vi "Main.vi"(7 "sweep rate, /min":dbl=0.2, 8 "sweep to:":dbl=4.0, 9 "sweep":T8(radio)=enum."2636a_smub") -> ()   [LabVIEW 2021] (continued)
                      # "we are  measuring 2182A 3 channel 1 (2182A_3_ch1)"
                      n2137 = local read "2182A 3 addr"() -> (w2872:u8)
                      n2138 = Number To Decimal String(number=w2872) -> (decimal integer string=w2871:string)  [unwired: 1 in]
                      n2139 = GPIB Write(0:w2871, 1:":SENSe:DATA:FRES?") -> (6:w2876:errorcluster)  [unwired: 3 in, 1 out]
                      n2140 = GPIB Read(0:w2871, 1:200, 3:w2876) -> (5:w2870:string)  [unwired: 2 in, 2 out]
                      n2141 = Fract/Exp String To Number(string=w2870) -> (number=w2874:dbl)  [unwired: 3 in, 1 out]
                      n2142 = Build Array (concatenate)(w2878, w2874) -> (w2877:dbl[])
                    }
                  }
                  n2143 = property on="data" class="Arr (strict)"("Value"=w2868) -> ()  [unwired: 2 in, 2 out]
                }
                frame #21 {
                  # "check if 2nd channel \non Keithley 2182A 3\nis to be measured"
                  n2144 = property on="data" class="Arr (strict)"() -> ("Value"=w2880:dbl[])  [unwired: 2 in, 2 out]
                  n2145 = local read "2182A 3 ch2"() -> (w2879:bool)
                  n2146 = case shown="True" w2879 {
                    tunnel: w2880 -> [w2882 w2895]
                    tunnel: [w2882 w2894] -> w2881
                    frame False {
                      # "we are not measuring 2182A 3 channel 2 (2182A_3_ch2)"
                    }
                    frame True {
                      # "switching to channel 2 and then\nback to channel 1"
                      # "we are  measuring 2182A 3 channel 2 (2182A_3_ch2)"
                      n2147 = local read "2182A 3 addr"() -> (w2889:u8)
                      n2148 = Number To Decimal String(number=w2889) -> (decimal integer string=w2884:string)  [unwired: 1 in]
                      n2149 = GPIB Write(0:w2884, 1:":SENSe:CHAN 2") -> (6:w2886:errorcluster)  [unwired: 3 in, 1 out]
                      n2150 = GPIB Write(0:w2884, 1:":SENSe:DATA:FRES?", 3:w2886) -> (6:w2893:errorcluster)  [unwired: 2 in, 1 out]
                      n2151 = GPIB Read(0:w2884, 1:200, 3:w2893) -> (5:w2888:string, 7:w2885:errorcluster)  [unwired: 2 in, 1 out]
                      n2152 = GPIB Write(0:w2884, 1:":SENSe:CHAN 1", 3:w2885) -> ()  [unwired: 2 in, 2 out]
                      n2153 = Fract/Exp String To Number(string=w2888) -> (number=w2891:dbl)  [unwired: 3 in, 1 out]
                      n2154 = Build Array (concatenate)(w2895, w2891) -> (w2894:dbl[])
                    }
                  }
                  n2155 = property on="data" class="Arr (strict)"("Value"=w2881) -> ()  [unwired: 2 in, 2 out]
                }
                frame #22 {
                  # "check if 1st channel \non Keithley 2182A 4\nis to be measured"
                  n2156 = property on="data" class="Arr (strict)"() -> ("Value"=w2897:dbl[])  [unwired: 2 in, 2 out]
                  n2157 = local read "2182A 4 ch1"() -> (w2896:bool)
                  n2158 = case shown="True" w2896 {
                    tunnel: w2897 -> [w2899 w2908]
                    tunnel: [w2899 w2907] -> w2898
                    frame False {
                      # "we are not measuring 2182A 4 channel 1 (2182A_4_ch1)"
                    }
                    frame True {
                      # "we are  measuring 2182A 4 channel 1 (2182A_4_ch1)"
                      n2159 = local read "2182A 4 addr"() -> (w2902:u8)
                      n2160 = Number To Decimal String(number=w2902) -> (decimal integer string=w2901:string)  [unwired: 1 in]
                      n2161 = GPIB Write(0:w2901, 1:":SENSe:DATA:FRES?") -> (6:w2906:errorcluster)  [unwired: 3 in, 1 out]
                      n2162 = GPIB Read(0:w2901, 1:200, 3:w2906) -> (5:w2900:string)  [unwired: 2 in, 2 out]
                      n2163 = Fract/Exp String To Number(string=w2900) -> (number=w2904:dbl)  [unwired: 3 in, 1 out]
                      n2164 = Build Array (concatenate)(w2908, w2904) -> (w2907:dbl[])
                    }
                  }
                  n2165 = property on="data" class="Arr (strict)"("Value"=w2898) -> ()  [unwired: 2 in, 2 out]
                }
                frame #23 {
                  # "check if 2nd channel \non Keithley 2182A 4\nis to be measured"
                  n2166 = property on="data" class="Arr (strict)"() -> ("Value"=w2910:dbl[])  [unwired: 2 in, 2 out]
                  n2167 = local read "2182A 4 ch2"() -> (w2909:bool)
                  n2168 = case shown="False" w2909 {
                    tunnel: w2910 -> [w2912 w2925]
                    tunnel: [w2912 w2924] -> w2911
                    frame False {
                      # "we are not measuring 2182A 4 channel 2 (2182A_4_ch2)"
                    }
                    frame True {
                      # "switching to channel 2 and then\nback to channel 1"
                      # "we are  measuring 2182A 4 channel 2 (2182A_4_ch2)"
                      n2169 = local read "2182A 4 addr"() -> (w2919:u8)
                      n2170 = Number To Decimal String(number=w2919) -> (decimal integer string=w2914:string)  [unwired: 1 in]
                      n2171 = GPIB Write(0:w2914, 1:":SENSe:CHAN 2") -> (6:w2916:errorcluster)  [unwired: 3 in, 1 out]
                      n2172 = GPIB Write(0:w2914, 1:":SENSe:DATA:FRES?", 3:w2916) -> (6:w2923:errorcluster)  [unwired: 2 in, 1 out]
                      n2173 = GPIB Read(0:w2914, 1:200, 3:w2923) -> (5:w2918:string, 7:w2915:errorcluster)  [unwired: 2 in, 1 out]
                      n2174 = GPIB Write(0:w2914, 1:":SENSe:CHAN 1", 3:w2915) -> ()  [unwired: 2 in, 2 out]
                      n2175 = Fract/Exp String To Number(string=w2918) -> (number=w2921:dbl)  [unwired: 3 in, 1 out]
                      n2176 = Build Array (concatenate)(w2925, w2921) -> (w2924:dbl[])
                    }
                  }
                  n2177 = property on="data" class="Arr (strict)"("Value"=w2911) -> ()  [unwired: 2 in, 2 out]
                }
                frame #24 {
                  # "check if voltage on\nKeithley 2636A smua\nis to be measured"
                  n2178 = local read "2636A smua meas v"() -> (w2926:bool)
                  n2179 = property on="data" class="Arr (strict)"() -> ("Value"=w2927:dbl[])  [unwired: 2 in, 2 out]
                  n2180 = case shown="True" w2926 {
                    tunnel: w2927 -> [w2929 w2935]
                    tunnel: [w2929 w2934] -> w2928
                    frame False {
                      # "we are not measuring voltage on 2636A smua (2636A_smua_v)"
                    }
                    frame True {
                      # "we are  measuring voltage on 2636A smua (2636A_smua_v)"
                      n2181 = local read "2614A addr"() -> (w2930:refnum<visa-resource-name>)
                      n2182 = call "SinglePointMeasurement.vi"("Measure"=Measure."Voltage", "Channel"=Channel."a", "VISA resource name 2"=w2930) -> ("Measuremet"=w2932:dbl)  [unwired: 3 in, 4 out]
                      n2183 = Build Array (concatenate)(w2935, w2932) -> (w2934:dbl[])
                    }
                  }
                  n2184 = property on="data" class="Arr (strict)"("Value"=w2928) -> ()  [unwired: 2 in, 2 out]
                }
                frame #25 {
                  # "check if current on\nKeithley 2636A smua\nis to be measured"
                  n2185 = local read "2636A smua meas i"() -> (w2936:bool)
                  n2186 = property on="data" class="Arr (strict)"() -> ("Value"=w2937:dbl[])  [unwired: 2 in, 2 out]
                  n2187 = case shown="True" w2936 {
                    tunnel: w2937 -> [w2939 w2942]
                    tunnel: [w2939 w2941] -> w2938
                    frame False {
                      # "we are not measuring current on 2636A smua (2636A_smua_i)"
                    }
                    frame True {
                      # "we are  measuring current on 2636A smua (2636A_smua_i)"
                      n2188 = stacked-sequence {
                        tunnel: [_ w2951] -> w2940
                        frame #0 {
                          n2189 = local read "auto\nrange A"() -> (w2946:bool)
                          n2190 = local read "2614A addr"() -> (w2949:refnum<visa-resource-name>)
                          n2191 = Select(t="smua.AUTORANGE_ON", s=w2946, f="smua.AUTORANGE_OFF") -> (s? t:f=w2944:string)
                          n2192 = Concatenate Strings("smua.measure.autorangei = ", w2944) -> (w2943:string)
                          n2193 = VISA Write(VISA resource name=w2949, write buffer=w2943) -> ()  [unwired: 1 in, 3 out]
                        }
                        frame #1 {
                          n2194 = local read "2614A addr"() -> (w2953:refnum<visa-resource-name>)
                          n2195 = call "SinglePointMeasurement.vi"("Measure"=Measure."Current", "Channel"=Channel."a", "VISA resource name 2"=w2953) -> ("Measuremet"=w2951:dbl)  [unwired: 3 in, 4 out]
                        }
                      }
                      n2196 = Build Array (concatenate)(w2942, w2940) -> (w2941:dbl[])
                    }
                  }
                  n2197 = property on="data" class="Arr (strict)"("Value"=w2938) -> ()  [unwired: 2 in, 2 out]
                }
                frame #26 {
                  # "check if voltage on\nKeithley 2636A smub\nis to be measured"
                  n2198 = local read "2636A smub meas v"() -> (w2954:bool)
                  n2199 = property on="data" class="Arr (strict)"() -> ("Value"=w2955:dbl[])  [unwired: 2 in, 2 out]
                  n2200 = case shown="True" w2954 {
                    tunnel: w2955 -> [w2957 w2963]
                    tunnel: [w2957 w2962] -> w2956
                    frame False {
                      # "we are not measuring voltage on 2636A smub (2636A_smub_v)"
                    }
                    frame True {
                      # "we are  measuring voltage on 2636A smub (2636A_smub_v)"
                      n2201 = local read "2614A addr"() -> (w2961:refnum<visa-resource-name>)
                      n2202 = call "SinglePointMeasurement.vi"("Measure"=Measure."Voltage", "Channel"=Channel."b", "VISA resource name 2"=w2961) -> ("Measuremet"=w2959:dbl)  [unwired: 3 in, 4 out]
                      n2203 = Build Array (concatenate)(w2963, w2959) -> (w2962:dbl[])
                    }
                  }
                  n2204 = property on="data" class="Arr (strict)"("Value"=w2956) -> ()  [unwired: 2 in, 2 out]
                }
                frame #27 {
                  # "check if current on\nKeithley 2636A smub\nis to be measured"
                  n2205 = local read "2636A smub meas i"() -> (w2964:bool)
                  n2206 = property on="data" class="Arr (strict)"() -> ("Value"=w2965:dbl[])  [unwired: 2 in, 2 out]
                  n2207 = case shown="True" w2964 {
                    tunnel: w2965 -> [w2967 w2970]
                    tunnel: [w2967 w2969] -> w2966
                    frame False {
                      # "we are not measuring current on 2636A smub (2636A_smub_i)"
                    }
                    frame True {
                      # "we are  measuring current on 2636A smub (2636A_smub_i)"
                      n2208 = stacked-sequence {
                        tunnel: [_ w2979] -> w2968
                        frame #0 {
                          n2209 = local read "auto\nrange B"() -> (w2974:bool)
                          n2210 = local read "2614A addr"() -> (w2977:refnum<visa-resource-name>)
                          n2211 = Select(t="smub.AUTORANGE_ON", s=w2974, f="smub.AUTORANGE_OFF") -> (s? t:f=w2972:string)
                          n2212 = Concatenate Strings("smub.measure.autorangei = ", w2972) -> (w2971:string)
                          n2213 = VISA Write(VISA resource name=w2977, write buffer=w2971) -> ()  [unwired: 1 in, 3 out]
                        }
                        frame #1 {
                          n2214 = local read "2614A addr"() -> (w2981:refnum<visa-resource-name>)
                          n2215 = call "SinglePointMeasurement.vi"("Measure"=Measure."Current", "Channel"=Channel."b", "VISA resource name 2"=w2981) -> ("Measuremet"=w2979:dbl)  [unwired: 3 in, 4 out]
                        }
                      }
                      n2216 = Build Array (concatenate)(w2970, w2968) -> (w2969:dbl[])
                    }
                  }
                  n2217 = property on="data" class="Arr (strict)"("Value"=w2966) -> ()  [unwired: 2 in, 2 out]
                }
                frame #28 {
                  # "check if time\nis to be measured"
                  n2218 = property on="data" class="Arr (strict)"() -> ("Value"=w2984:dbl[])  [unwired: 2 in, 2 out]
                  n2219 = local read "measure time"() -> (w2983:bool)
                  n2220 = case shown="True" w2983 {
                    tunnel: w2984 -> [w2986 w2992]
                    tunnel: [w2986 w2991] -> w2985
                    tunnel: w2982 -> [_ w2989]
                    frame False {
                      # "we are not measuring time"
                    }
                    frame True {
                      # "seconds from the beginning of month"
                      # "we are  measuring time"
                      n2221 = call "timeInSeconds.vi"() -> ("Numeric"=w2990:dbl, "current time"=w2987:timestamp)  [unwired: 2 in]
                      n2222 = property on="current time" class="AbsTime (strict)"("Value"=w2987) -> ()  [unwired: 2 in, 2 out]
                      n2223 = Subtract(x=w2990, y=w2989) -> (x-y=w2988:dbl)
                      n2224 = Build Array (concatenate)(w2992, w2988) -> (w2991:dbl[])
                    }
                  }
                  n2225 = property on="data" class="Arr (strict)"("Value"=w2985) -> ()  [unwired: 2 in, 2 out]
                }
                frame #29 {
                  n2226 = local read "MagnetField"() -> (w2993:bool)
                  n2227 = property on="data" class="Arr (strict)"() -> ("Value"=w2994:dbl[])  [unwired: 2 in, 2 out]
                  n2228 = case shown="True" w2993 {
                    tunnel: w2994 -> [w2996 w2999]
                    tunnel: [w2996 w2998] -> w2995
                    frame False {
                      # "we are not Measuring magnetic field on IPS120-0"
                    }
                    frame True {
                      # "Measure magnetic field on Teslatron_iPS_Field"
                      n2229 = call "TRITON_Read Field.vi"() -> ("Measurement"=w2997:dbl)  [unwired: 2 in, 1 out]
                      n2230 = Build Array (concatenate)(w2999, w2997) -> (w2998:dbl[])
                    }
                  }
                  n2231 = property on="data" class="Arr (strict)"("Value"=w2995) -> ()  [unwired: 2 in, 2 out]
                }
                frame #30 {
                  n2232 = property on="data" class="Arr (strict)"() -> ("Value"=w3001:dbl[])  [unwired: 2 in, 2 out]
                  n2233 = property on="Magnet_T" class="Bool (strict)"() -> ("Value"=w3000:bool)  [unwired: 2 in, 2 out]
                  n2234 = case shown="True" w3000 {
                    tunnel: w3001 -> [w3003 w3007]
                    tunnel: [w3003 w3006] -> w3002
                    frame False {
                      # "we are not Measuring magnetic field on IPS120-0"
                    }
                    frame True {
                      # "Measure magnetic_T on Teslatron"
                      n2235 = call "TRITON_Read Temperature.vi"("Channel"=13 ("Ch2")) -> ("Measuremet"=w3004:dbl)  [unwired: 1 in, 1 out]
                      n2236 = Build Array (concatenate)(w3007, w3004) -> (w3006:dbl[])
                    }
                  }
                  n2237 = property on="data" class="Arr (strict)"("Value"=w3002) -> ()  [unwired: 2 in, 2 out]
                }
                frame #31 {
                  n2238 = property on="data" class="Arr (strict)"() -> ("Value"=w3009:dbl[])  [unwired: 2 in, 2 out]
                  n2239 = property on="PT1" class="Bool (strict)"() -> ("Value"=w3008:bool)  [unwired: 2 in, 2 out]
                  n2240 = case shown="True" w3008 {
                    tunnel: w3009 -> [w3011 w3015]
                    tunnel: [w3011 w3014] -> w3010
                    frame False {
                      # "we are not Measuring magnetic field on IPS120-0"
                    }
                    frame True {
                      # "Measure  SH_T on Teslatron"
                      n2241 = call "TRITON_Read Temperature.vi"("Channel"=7 ("Ch2")) -> ("Measuremet"=w3012:dbl)  [unwired: 1 in, 1 out]
                      n2242 = Build Array (concatenate)(w3015, w3012) -> (w3014:dbl[])
                    }
                  }
                  n2243 = property on="data" class="Arr (strict)"("Value"=w3010) -> ()  [unwired: 2 in, 2 out]
                }
                frame #32 {
                  # "check if current \non 2461 SouceMeter\nis to be measured"
                  n2244 = property on="data" class="Arr (strict)"() -> ("Value"=w3017:dbl[])  [unwired: 2 in, 2 out]
                  n2245 = property on="MC_RuO2" class="Bool (strict)"() -> ("Value"=w3016:bool)  [unwired: 2 in, 2 out]
                  n2246 = case shown="True" w3016 {
                    tunnel: w3017 -> [w3019 w3023]
                    tunnel: [w3019 w3022] -> w3018
                    frame False {
                      # "we are not measuring 2461, voltage (2461_meas_v)"
                    }
                    frame True {
                      # "we are  measuring 2461, voltage (2461_meas_v)"
                      n2247 = call "TRITON_Read Temperature.vi"("Channel"=8 ("Ch2")) -> ("Measuremet"=w3020:dbl)  [unwired: 1 in, 1 out]
                      n2248 = Build Array (concatenate)(w3023, w3020) -> (w3022:dbl[])
                    }
                  }
                  n2249 = property on="data" class="Arr (strict)"("Value"=w3018) -> ()  [unwired: 2 in, 2 out]
                }
                frame #33 {
                  # "check if current \non 2461 SouceMeter\nis to be measured"
                  n2250 = property on="data" class="Arr (strict)"() -> ("Value"=w3025:dbl[])  [unwired: 2 in, 2 out]
                  n2251 = property on="Still" class="Bool (strict)"() -> ("Value"=w3024:bool)  [unwired: 2 in, 2 out]
                  n2252 = case shown="True" w3024 {
                    tunnel: w3025 -> [w3027 w3031]
                    tunnel: [w3027 w3030] -> w3026
                    frame False {
                      # "we are not measuring 2461, voltage (2461_meas_v)"
                    }
                    frame True {
                      # "we are  measuring 2461, voltage (2461_meas_v)"
                      n2253 = call "TRITON_Read Temperature.vi"("Channel"=3 ("Ch2")) -> ("Measuremet"=w3028:dbl)  [unwired: 1 in, 1 out]
                      n2254 = Build Array (concatenate)(w3031, w3028) -> (w3030:dbl[])
                    }
                  }
                  n2255 = property on="data" class="Arr (strict)"("Value"=w3026) -> ()  [unwired: 2 in, 2 out]
                }
                frame #34 {
                  # "check if current \non 2461 SouceMeter\nis to be measured"
                  n2256 = property on="data" class="Arr (strict)"() -> ("Value"=w3033:dbl[])  [unwired: 2 in, 2 out]
                  n2257 = property on="Cold_Plate" class="Bool (strict)"() -> ("Value"=w3032:bool)  [unwired: 2 in, 2 out]
                  n2258 = case shown="True" w3032 {
                    tunnel: w3033 -> [w3035 w3039]
                    tunnel: [w3035 w3038] -> w3034
                    frame False {
                      # "we are not measuring 2461, voltage (2461_meas_v)"
                    }
                    frame True {
                      # "we are  measuring 2461, voltage (2461_meas_v)"
                      n2259 = call "TRITON_Read Temperature.vi"("Channel"=4 ("Ch2")) -> ("Measuremet"=w3036:dbl)  [unwired: 1 in, 1 out]
                      n2260 = Build Array (concatenate)(w3039, w3036) -> (w3038:dbl[])
                    }
                  }
                  n2261 = property on="data" class="Arr (strict)"("Value"=w3034) -> ()  [unwired: 2 in, 2 out]
                }
                frame #35 {
                  # "check if current \non 2461 SouceMeter\nis to be measured"
                  n2262 = property on="data" class="Arr (strict)"() -> ("Value"=w3041:dbl[])  [unwired: 2 in, 2 out]
                  n2263 = property on="PT2" class="Bool (strict)"() -> ("Value"=w3040:bool)  [unwired: 2 in, 2 out]
                  n2264 = case shown="True" w3040 {
                    tunnel: w3041 -> [w3043 w3047]
                    tunnel: [w3043 w3046] -> w3042
                    frame False {
                      # "we are not measuring 2461, voltage (2461_meas_v)"
                    }
                    frame True {
                      # "we are  measuring 2461, voltage (2461_meas_v)"
                      n2265 = call "TRITON_Read Temperature.vi"("Channel"=2 ("Ch2")) -> ("Measuremet"=w3044:dbl)  [unwired: 1 in, 1 out]
                      n2266 = Build Array (concatenate)(w3047, w3044) -> (w3046:dbl[])
                    }
                  }
                  n2267 = property on="data" class="Arr (strict)"("Value"=w3042) -> ()  [unwired: 2 in, 2 out]
                }
                frame #36 {
                  # "check if current \non 2461 SouceMeter\nis to be measured"
                  n2268 = property on="data" class="Arr (strict)"() -> ("Value"=w3049:dbl[])  [unwired: 2 in, 2 out]
                  n2269 = property on="MC_Cernox" class="Bool (strict)"() -> ("Value"=w3048:bool)  [unwired: 2 in, 2 out]
                  n2270 = case shown="True" w3048 {
                    tunnel: w3049 -> [w3051 w3055]
                    tunnel: [w3051 w3054] -> w3050
                    frame False {
                      # "we are not measuring 2461, voltage (2461_meas_v)"
                    }
                    frame True {
                      # "we are  measuring 2461, voltage (2461_meas_v)"
                      n2271 = call "TRITON_Read Temperature.vi"("Channel"=5 ("Ch2")) -> ("Measuremet"=w3052:dbl)  [unwired: 1 in, 1 out]
                      n2272 = Build Array (concatenate)(w3055, w3052) -> (w3054:dbl[])
                    }
                  }
                  n2273 = property on="data" class="Arr (strict)"("Value"=w3050) -> ()  [unwired: 2 in, 2 out]
                }
                frame #37 {
                  # "check if current \non 2461 SouceMeter\nis to be measured"
                  n2274 = property on="2461_meas_v" class="Bool (strict)"() -> ("Value"=w3056:bool)  [unwired: 2 in, 2 out]
                  n2275 = property on="data" class="Arr (strict)"() -> ("Value"=w3057:dbl[])  [unwired: 2 in, 2 out]
                  n2276 = case shown="True" w3056 {
                    tunnel: w3057 -> [w3059 w3064]
                    tunnel: [w3059 w3063] -> w3058
                    frame False {
                      # "we are not measuring 2461, voltage (2461_meas_v)"
                    }
                    frame True {
                      # "we are  measuring 2461, voltage (2461_meas_v)"
                      n2277 = property on="2461_addr_sweep" class="VISAName"() -> ("Value"=w3061:refnum<visa-resource-name>)  [unwired: 2 in, 2 out]
                      n2278 = call <instrlib>:"Read (Single Point).vi"("VISA resource name"=w3061) -> ("Data out"=w3060:string)  [unwired: 12 in, 2 out]
                      n2279 = Fract/Exp String To Number(string=w3060) -> (number=w3062:dbl)  [unwired: 3 in, 1 out]
                      n2280 = Build Array (concatenate)(w3064, w3062) -> (w3063:dbl[])
                    }
                  }
                  n2281 = property on="data" class="Arr (strict)"("Value"=w3058) -> ()  [unwired: 2 in, 2 out]
                }
                frame #38 {
                  # "check if current \non 2461 SouceMeter\nis to be measured"
                  n2282 = property on="2461_meas_i" class="Bool (strict)"() -> ("Value"=w3065:bool)  [unwired: 2 in, 2 out]
                  n2283 = property on="data" class="Arr (strict)"() -> ("Value"=w3066:dbl[])  [unwired: 2 in, 2 out]
                  n2284 = case shown="True" w3065 {
                    tunnel: w3066 -> [w3068 w3072]
                    tunnel: [w3068 w3071] -> w3067
                    frame False {
                      # "we are not measuring 2461, voltage (2461_meas_v)"
                    }
                    frame True {
                      # "we are  measuring 2461, curent (2461_meas_i)"
                      n2285 = property on="2461_addr_sweep" class="VISAName"() -> ("Value"=w3070:refnum<visa-resource-name>)  [unwired: 2 in, 2 out]
                      n2286 = call <instrlib>:"Get Source Level.vi"("VISA resource name"=w3070) -> ("Current Level Out"=w3069:dbl)  [unwired: 7 in, 3 out]
                      n2287 = Build Array (concatenate)(w3072, w3069) -> (w3071:dbl[])
                    }
                  }
                  n2288 = property on="data" class="Arr (strict)"("Value"=w3067) -> ()  [unwired: 2 in, 2 out]
                }
                frame #39 {
                  # "Record Step Value \nif it is mapping"
                  n2289 = property on="Linetrace or Mapping?" class="Bool (strict)"() -> ("Value"=w3074:bool)  [unwired: 2 in, 2 out]
                  n2290 = property on="data" class="Arr (strict)"() -> ("Value"=w3075:dbl[])  [unwired: 2 in, 2 out]
                  n2291 = case shown="True" w3074 {
                    tunnel: w3075 -> [w3076 w3079]
                    tunnel: [w3076 w3078] -> w3073
                    frame False {
                      # "We are not recording Step Value if it is linetrace"
                    }
                    frame True {
                      # "We are recording Step Value if it is mapping"
                      n2292 = property on="Current Step Value" class="DigNum (strict)"() -> ("Value"=w3077:dbl)  [unwired: 2 in, 2 out]
                      n2293 = Build Array (concatenate)(w3079, w3077) -> (w3078:dbl[])
                    }
                  }
                  n2294 = property on="data" class="Arr (strict)"("Value"=w3073) -> ()  [unwired: 2 in, 2 out]
                }
                frame #40 {
                  # "Record Step Value \nif it is mapping"
                  n2295 = property on="HyperLoop" class="Bool (strict)"() -> ("Value"=w3080:bool)  [unwired: 2 in, 2 out]
                  n2296 = property on="data" class="Arr (strict)"() -> ("Value"=w3082:dbl[])  [unwired: 2 in, 2 out]
                  n2297 = case shown="True" w3080 {
                    tunnel: w3082 -> [w3083 w3086]
                    tunnel: [w3083 w3085] -> w3081
                    frame False {
                      # "We are not recording Step Value if it is linetrace"
                    }
                    frame True {
                      # "We are recording Step Value if it is mapping"
                      n2298 = property on="Current Hyper Value" class="DigNum (strict)"() -> ("Value"=w3084:dbl)  [unwired: 2 in, 2 out]
                      n2299 = Build Array (concatenate)(w3086, w3084) -> (w3085:dbl[])
                    }
                  }
                  n2300 = property on="data" class="Arr (strict)"("Value"=w3081) -> ()  [unwired: 2 in, 2 out]
                }
                frame #41 {
                  # "Record Step Value \nif it is mapping"
                  n2301 = property on="SuperHyper" class="Bool (strict)"() -> ("Value"=w3087:bool)  [unwired: 2 in, 2 out]
                  n2302 = property on="data" class="Arr (strict)"() -> ("Value"=w3089:dbl[])  [unwired: 2 in, 2 out]
                  n2303 = case shown="True" w3087 {
                    tunnel: w3089 -> [w3090 w3093]
                    tunnel: [w3090 w3092] -> w3088
                    frame False {
                      # "We are not recording Step Value if it is linetrace"
                    }
                    frame True {
                      # "We are recording SuperHyper_step if it is mapping"
                      n2304 = property on="Current SuperHyper Value" class="DigNum (strict)"() -> ("Value"=w3091:dbl)  [unwired: 2 in, 2 out]
                      n2305 = Build Array (concatenate)(w3093, w3091) -> (w3092:dbl[])
                    }
                  }
                  n2306 = property on="data" class="Arr (strict)"("Value"=w3088) -> ()  [unwired: 2 in, 2 out]
                }
                frame #42 {
                  # "Measure MFLI_V if \nit is checked"
                  n2307 = property on="MFLI1_d0" class="Bool (strict)"() -> ("Value"=w3094:bool)  [unwired: 2 in, 2 out]
                  n2308 = property on="data" class="Arr (strict)"() -> ("Value"=w3096:dbl[])  [unwired: 2 in, 2 out]
                  n2309 = case shown="True" w3094 {
                    tunnel: w3096 -> [w3097 w3102]
                    tunnel: [w3097 w3101] -> w3095
                    frame False {
                      # "We are not recording Step Value if it is linetrace"
                    }
                    frame True {
                      n2310 = flat-sequence {
                        tunnel: [w3106] -> w3100
                        tunnel: [w3105] -> w3099
                        tunnel: [w3104] -> w3098
                        frame #0 {
                          n2311 = property on="HandleOut" class="Clust (strict)"() -> ("Value"=w3108:T1)  [unwired: 2 in, 2 out]
                          n2312 = call "MFLIcontrol.vi"("MFLI function"=MFLIcommand."measure XY on demod0", "handle in"=w3108) -> ("Demod Sample Out 2"=w3103:T20)  [unwired: 5 in, 4 out]
                          n2313 = Unbundle(w3103) -> ("X (Vrms)"=w3106:dbl, "Y (Vrms)"=w3105:dbl, "Freq (Hz)"=w3104:dbl)  [unwired: 6 out]
                        }
                      }
                      n2314 = Build Array (concatenate)(w3102, w3100, w3099, w3098) -> (w3101:dbl[])
                    }
                  }
                  n2315 = property on="data" class="Arr (strict)"("Value"=w3095) -> ()  [unwired: 2 in, 2 out]
                }
                frame #43 {
                  # "Measure MFLI_V if \nit is checked"
                  n2316 = property on="MFLI2_d0" class="Bool (strict)"() -> ("Value"=w3109:bool)  [unwired: 2 in, 2 out]
                  n2317 = property on="data" class="Arr (strict)"() -> ("Value"=w3111:dbl[])  [unwired: 2 in, 2 out]
                  n2318 = case shown="True" w3109 {
                    tunnel: w3111 -> [w3112 w3117]
                    tunnel: [w3112 w3116] -> w3110
                    frame False {
                      # "We are not recording Step Value if it is linetrace"
                    }
                    frame True {
                      n2319 = flat-sequence {
                        tunnel: [w3121] -> w3115
                        tunnel: [w3120] -> w3114
                        tunnel: [w3119] -> w3113
                        frame #0 {
                          n2320 = property on="HandleOut 2" class="Clust (strict)"() -> ("Value"=w3123:T21)  [unwired: 2 in, 2 out]
                          n2321 = call "MFLIcontrol.vi"("MFLI function"=MFLIcommand."measure XY on demod0", "handle in"=w3123) -> ("Demod Sample Out 2"=w3118:T20)  [unwired: 5 in, 4 out]
                          n2322 = Unbundle(w3118) -> ("X (Vrms)"=w3121:dbl, "Y (Vrms)"=w3120:dbl, "Freq (Hz)"=w3119:dbl)  [unwired: 6 out]
                        }
                      }
                      n2323 = Build Array (concatenate)(w3117, w3115, w3114, w3113) -> (w3116:dbl[])
                    }
                  }
                  n2324 = property on="data" class="Arr (strict)"("Value"=w3110) -> ()  [unwired: 2 in, 2 out]
                }
                frame #44 {
                  # "Measure MFLI_V if \nit is checked"
                  n2325 = property on="MFLI3_d0" class="Bool (strict)"() -> ("Value"=w3124:bool)  [unwired: 2 in, 2 out]
                  n2326 = property on="data" class="Arr (strict)"() -> ("Value"=w3126:dbl[])  [unwired: 2 in, 2 out]
                  n2327 = case shown="True" w3124 {
                    tunnel: w3126 -> [w3127 w3132]
                    tunnel: [w3127 w3131] -> w3125
                    frame False {
                      # "We are not recording Step Value if it is linetrace"
                    }
                    frame True {
                      n2328 = flat-sequence {
                        tunnel: [w3136] -> w3130
                        tunnel: [w3135] -> w3129
                        tunnel: [w3134] -> w3128
                        frame #0 {
                          n2329 = property on="HandleOut 3" class="Clust (strict)"() -> ("Value"=w3138:T21)  [unwired: 2 in, 2 out]
                          n2330 = call "MFLIcontrol.vi"("MFLI function"=MFLIcommand."measure XY on demod0", "handle in"=w3138) -> ("Demod Sample Out 2"=w3133:T20)  [unwired: 5 in, 4 out]
                          n2331 = Unbundle(w3133) -> ("X (Vrms)"=w3136:dbl, "Y (Vrms)"=w3135:dbl, "Freq (Hz)"=w3134:dbl)  [unwired: 6 out]
                        }
                      }
                      n2332 = Build Array (concatenate)(w3132, w3130, w3129, w3128) -> (w3131:dbl[])
                    }
                  }
                  n2333 = property on="data" class="Arr (strict)"("Value"=w3125) -> ()  [unwired: 2 in, 2 out]
                }
                frame #45 {
                  # "Measure MFLI_V if \nit is checked"
                  n2334 = property on="MFLI4_d0" class="Bool (strict)"() -> ("Value"=w3139:bool)  [unwired: 2 in, 2 out]
                  n2335 = property on="data" class="Arr (strict)"() -> ("Value"=w3141:dbl[])  [unwired: 2 in, 2 out]
                  n2336 = case shown="True" w3139 {
                    tunnel: w3141 -> [w3142 w3147]
                    tunnel: [w3142 w3146] -> w3140
                    frame False {
                      # "We are not recording Step Value if it is linetrace"
                    }
                    frame True {
                      n2337 = flat-sequence {
                        tunnel: [w3151] -> w3145
                        tunnel: [w3150] -> w3144
                        tunnel: [w3149] -> w3143
                        frame #0 {
                          n2338 = property on="HandleOut 4" class="Clust (strict)"() -> ("Value"=w3153:T21)  [unwired: 2 in, 2 out]
                          n2339 = call "MFLIcontrol.vi"("MFLI function"=MFLIcommand."measure XY on demod0", "handle in"=w3153) -> ("Demod Sample Out 2"=w3148:T20)  [unwired: 5 in, 4 out]
                          n2340 = Unbundle(w3148) -> ("X (Vrms)"=w3151:dbl, "Y (Vrms)"=w3150:dbl, "Freq (Hz)"=w3149:dbl)  [unwired: 6 out]
                        }
                      }
                      n2341 = Build Array (concatenate)(w3147, w3145, w3144, w3143) -> (w3146:dbl[])
                    }
                  }
                  n2342 = property on="data" class="Arr (strict)"("Value"=w3140) -> ()  [unwired: 2 in, 2 out]
                }
                frame #46 {
                  # "Measure MFLI_I if \nit is checked"
                  n2343 = property on="MFLI1_d1" class="Bool (strict)"() -> ("Value"=w3154:bool)  [unwired: 2 in, 2 out]
                  n2344 = property on="data" class="Arr (strict)"() -> ("Value"=w3156:dbl[])  [unwired: 2 in, 2 out]
                  n2345 = case shown="True" w3154 {
                    tunnel: w3156 -> [w3157 w3162]
                    tunnel: [w3157 w3161] -> w3155
                    frame False {
                      # "We are not recording Step Value if it is linetrace"
                    }
                    frame True {
                      n2346 = flat-sequence {
                        tunnel: [w3165] -> w3160
                        tunnel: [w3164] -> w3159
                        tunnel: [w3163] -> w3158
                        frame #0 {
                          n2347 = property on="HandleOut" class="Clust (strict)"() -> ("Value"=w3168:T1)  [unwired: 2 in, 2 out]
                          n2348 = call "MFLIcontrol.vi"("MFLI function"=MFLIcommand."measure XY on demod1", "handle in"=w3168) -> ("Demod Sample Out 3"=w3166:T20)  [unwired: 5 in, 4 out]
                          n2349 = Unbundle(w3166) -> ("X (Vrms)"=w3165:dbl, "Y (Vrms)"=w3164:dbl, "Freq (Hz)"=w3163:dbl)  [unwired: 6 out]
                        }
                      }
                      n2350 = Build Array (concatenate)(w3162, w3160, w3159, w3158) -> (w3161:dbl[])
                    }
                  }
                  n2351 = property on="data" class="Arr (strict)"("Value"=w3155) -> ()  [unwired: 2 in, 2 out]
                }
                frame #47 {
                  # "Measure MFLI_I if \nit is checked"
                  n2352 = property on="MFLI2_d1" class="Bool (strict)"() -> ("Value"=w3169:bool)  [unwired: 2 in, 2 out]
                  n2353 = property on="data" class="Arr (strict)"() -> ("Value"=w3171:dbl[])  [unwired: 2 in, 2 out]
                  n2354 = case shown="True" w3169 {
                    tunnel: w3171 -> [w3172 w3177]
                    tunnel: [w3172 w3176] -> w3170
                    frame False {
                      # "We are not recording Step Value if it is linetrace"
                    }
                    frame True {
                      n2355 = flat-sequence {
                        tunnel: [w3180] -> w3175
                        tunnel: [w3179] -> w3174
                        tunnel: [w3178] -> w3173
                        frame #0 {
                          n2356 = property on="HandleOut 2" class="Clust (strict)"() -> ("Value"=w3183:T21)  [unwired: 2 in, 2 out]
                          n2357 = call "MFLIcontrol.vi"("MFLI function"=MFLIcommand."measure XY on demod1", "handle in"=w3183) -> ("Demod Sample Out 3"=w3181:T20)  [unwired: 5 in, 4 out]
                          n2358 = Unbundle(w3181) -> ("X (Vrms)"=w3180:dbl, "Y (Vrms)"=w3179:dbl, "Freq (Hz)"=w3178:dbl)  [unwired: 6 out]
                        }
                      }
                      n2359 = Build Array (concatenate)(w3177, w3175, w3174, w3173) -> (w3176:dbl[])
                    }
                  }
                  n2360 = property on="data" class="Arr (strict)"("Value"=w3170) -> ()  [unwired: 2 in, 2 out]
                }
                frame #48 {
                  # "Measure MFLI_I if \nit is checked"
                  n2361 = property on="MFLI3_d1" class="Bool (strict)"() -> ("Value"=w3184:bool)  [unwired: 2 in, 2 out]
                  n2362 = property on="data" class="Arr (strict)"() -> ("Value"=w3186:dbl[])  [unwired: 2 in, 2 out]
                  n2363 = case shown="True" w3184 {
                    tunnel: w3186 -> [w3187 w3192]
                    tunnel: [w3187 w3191] -> w3185
                    frame False {
                      # "We are not recording Step Value if it is linetrace"
                    }
                    frame True {
                      n2364 = flat-sequence {
                        tunnel: [w3195] -> w3190
                        tunnel: [w3194] -> w3189
                        tunnel: [w3193] -> w3188
                        frame #0 {
                          n2365 = property on="HandleOut 3" class="Clust (strict)"() -> ("Value"=w3198:T21)  [unwired: 2 in, 2 out]
                          n2366 = call "MFLIcontrol.vi"("MFLI function"=MFLIcommand."measure XY on demod1", "handle in"=w3198) -> ("Demod Sample Out 3"=w3196:T20)  [unwired: 5 in, 4 out]
                          n2367 = Unbundle(w3196) -> ("X (Vrms)"=w3195:dbl, "Y (Vrms)"=w3194:dbl, "Freq (Hz)"=w3193:dbl)  [unwired: 6 out]
                        }
                      }
                      n2368 = Build Array (concatenate)(w3192, w3190, w3189, w3188) -> (w3191:dbl[])
                    }
                  }
                  n2369 = property on="data" class="Arr (strict)"("Value"=w3185) -> ()  [unwired: 2 in, 2 out]
                }
                frame #49 {
                  # "Measure MFLI_I if \nit is checked"
                  n2370 = property on="MFLI4_d1" class="Bool (strict)"() -> ("Value"=w3199:bool)  [unwired: 2 in, 2 out]
                  n2371 = property on="data" class="Arr (strict)"() -> ("Value"=w3201:dbl[])  [unwired: 2 in, 2 out]
                  n2372 = case shown="True" w3199 {
                    tunnel: w3201 -> [w3202 w3207]
                    tunnel: [w3202 w3206] -> w3200
                    frame False {
                      # "We are not recording Step Value if it is linetrace"
                    }
                    frame True {
                      n2373 = flat-sequence {
                        tunnel: [w3210] -> w3205
                        tunnel: [w3209] -> w3204
                        tunnel: [w3208] -> w3203
                        frame #0 {
                          n2374 = property on="HandleOut 4" class="Clust (strict)"() -> ("Value"=w3213:T21)  [unwired: 2 in, 2 out]
                          n2375 = call "MFLIcontrol.vi"("MFLI function"=MFLIcommand."measure XY on demod1", "handle in"=w3213) -> ("Demod Sample Out 3"=w3211:T20)  [unwired: 5 in, 4 out]
                          n2376 = Unbundle(w3211) -> ("X (Vrms)"=w3210:dbl, "Y (Vrms)"=w3209:dbl, "Freq (Hz)"=w3208:dbl)  [unwired: 6 out]
                        }
                      }
                      n2377 = Build Array (concatenate)(w3207, w3205, w3204, w3203) -> (w3206:dbl[])
                    }
                  }
                  n2378 = property on="data" class="Arr (strict)"("Value"=w3200) -> ()  [unwired: 2 in, 2 out]
                }
                frame #50 {
                  # "Measure MFLI_I if \nit is checked"
                  n2379 = property on="MFLI1_d2" class="Bool (strict)"() -> ("Value"=w3214:bool)  [unwired: 2 in, 2 out]
                  n2380 = property on="data" class="Arr (strict)"() -> ("Value"=w3216:dbl[])  [unwired: 2 in, 2 out]
                  n2381 = case shown="True" w3214 {
                    tunnel: w3216 -> [w3217 w3222]
                    tunnel: [w3217 w3221] -> w3215
                    frame False {
                      # "We are not recording Step Value if it is linetrace"
                    }
                    frame True {
                      n2382 = flat-sequence {
                        tunnel: [w3225] -> w3220
                        tunnel: [w3224] -> w3219
                        tunnel: [w3223] -> w3218
                        frame #0 {
                          n2383 = property on="HandleOut" class="Clust (strict)"() -> ("Value"=w3228:T1)  [unwired: 2 in, 2 out]
                          n2384 = call "MFLIcontrol.vi"("MFLI function"=MFLIcommand."measure XY on demod2", "handle in"=w3228) -> ("Demod Sample Out 3"=w3226:T20)  [unwired: 5 in, 4 out]
                          n2385 = Unbundle(w3226) -> ("X (Vrms)"=w3225:dbl, "Y (Vrms)"=w3224:dbl, "Freq (Hz)"=w3223:dbl)  [unwired: 6 out]
                        }
                      }
                      n2386 = Build Array (concatenate)(w3222, w3220, w3219, w3218) -> (w3221:dbl[])
                    }
                  }
                  n2387 = property on="data" class="Arr (strict)"("Value"=w3215) -> ()  [unwired: 2 in, 2 out]
                }
                frame #51 {
                  # "Measure MFLI_I if \nit is checked"
                  n2388 = property on="MFLI2_d2" class="Bool (strict)"() -> ("Value"=w3229:bool)  [unwired: 2 in, 2 out]
                  n2389 = property on="data" class="Arr (strict)"() -> ("Value"=w3231:dbl[])  [unwired: 2 in, 2 out]
                  n2390 = case shown="True" w3229 {
                    tunnel: w3231 -> [w3232 w3237]
                    tunnel: [w3232 w3236] -> w3230
                    frame False {
                      # "We are not recording Step Value if it is linetrace"
                    }
                    frame True {
                      n2391 = flat-sequence {
                        tunnel: [w3240] -> w3235
                        tunnel: [w3239] -> w3234
                        tunnel: [w3238] -> w3233
                        frame #0 {
                          n2392 = property on="HandleOut 2" class="Clust (strict)"() -> ("Value"=w3243:T21)  [unwired: 2 in, 2 out]
                          n2393 = call "MFLIcontrol.vi"("MFLI function"=MFLIcommand."measure XY on demod2", "handle in"=w3243) -> ("Demod Sample Out 3"=w3241:T20)  [unwired: 5 in, 4 out]
                          n2394 = Unbundle(w3241) -> ("X (Vrms)"=w3240:dbl, "Y (Vrms)"=w3239:dbl, "Freq (Hz)"=w3238:dbl)  [unwired: 6 out]
                        }
                      }
                      n2395 = Build Array (concatenate)(w3237, w3235, w3234, w3233) -> (w3236:dbl[])
                    }
                  }
                  n2396 = property on="data" class="Arr (strict)"("Value"=w3230) -> ()  [unwired: 2 in, 2 out]
                }
                frame #52 {
                  # "Measure MFLI_I if \nit is checked"
                  n2397 = property on="MFLI3_d2" class="Bool (strict)"() -> ("Value"=w3244:bool)  [unwired: 2 in, 2 out]
                  n2398 = property on="data" class="Arr (strict)"() -> ("Value"=w3246:dbl[])  [unwired: 2 in, 2 out]
                  n2399 = case shown="True" w3244 {
                    tunnel: w3246 -> [w3247 w3252]
                    tunnel: [w3247 w3251] -> w3245
                    frame False {
                      # "We are not recording Step Value if it is linetrace"
                    }
                    frame True {
                      n2400 = flat-sequence {
                        tunnel: [w3255] -> w3250
                        tunnel: [w3254] -> w3249
                        tunnel: [w3253] -> w3248
                        frame #0 {
                          n2401 = property on="HandleOut 3" class="Clust (strict)"() -> ("Value"=w3258:T21)  [unwired: 2 in, 2 out]
                          n2402 = call "MFLIcontrol.vi"("MFLI function"=MFLIcommand."measure XY on demod2", "handle in"=w3258) -> ("Demod Sample Out 3"=w3256:T20)  [unwired: 5 in, 4 out]
                          n2403 = Unbundle(w3256) -> ("X (Vrms)"=w3255:dbl, "Y (Vrms)"=w3254:dbl, "Freq (Hz)"=w3253:dbl)  [unwired: 6 out]
                        }
                      }
                      n2404 = Build Array (concatenate)(w3252, w3250, w3249, w3248) -> (w3251:dbl[])
                    }
                  }
                  n2405 = property on="data" class="Arr (strict)"("Value"=w3245) -> ()  [unwired: 2 in, 2 out]
                }
                frame #53 {
                  # "Measure MFLI_I if \nit is checked"
                  n2406 = property on="MFLI4_d2" class="Bool (strict)"() -> ("Value"=w3259:bool)  [unwired: 2 in, 2 out]
                  n2407 = property on="data" class="Arr (strict)"() -> ("Value"=w3261:dbl[])  [unwired: 2 in, 2 out]
                  n2408 = case shown="True" w3259 {
                    tunnel: w3261 -> [w3262 w3267]
                    tunnel: [w3262 w3266] -> w3260
                    frame False {
                      # "We are not recording Step Value if it is linetrace"
                    }
                    frame True {
                      n2409 = flat-sequence {
                        tunnel: [w3270] -> w3265
                        tunnel: [w3269] -> w3264
                        tunnel: [w3268] -> w3263
                        frame #0 {
                          n2410 = property on="HandleOut 4" class="Clust (strict)"() -> ("Value"=w3273:T21)  [unwired: 2 in, 2 out]
                          n2411 = call "MFLIcontrol.vi"("MFLI function"=MFLIcommand."measure XY on demod2", "handle in"=w3273) -> ("Demod Sample Out 3"=w3271:T20)  [unwired: 5 in, 4 out]
                          n2412 = Unbundle(w3271) -> ("X (Vrms)"=w3270:dbl, "Y (Vrms)"=w3269:dbl, "Freq (Hz)"=w3268:dbl)  [unwired: 6 out]
                        }
                      }
                      n2413 = Build Array (concatenate)(w3267, w3265, w3264, w3263) -> (w3266:dbl[])
                    }
                  }
                  n2414 = property on="data" class="Arr (strict)"("Value"=w3260) -> ()  [unwired: 2 in, 2 out]
                }
                frame #54 {
                  # "Measure MFLI_I if \nit is checked"
                  n2415 = property on="MFLI1_d3" class="Bool (strict)"() -> ("Value"=w3274:bool)  [unwired: 2 in, 2 out]
                  n2416 = property on="data" class="Arr (strict)"() -> ("Value"=w3276:dbl[])  [unwired: 2 in, 2 out]
                  n2417 = case shown="True" w3274 {
                    tunnel: w3276 -> [w3277 w3282]
                    tunnel: [w3277 w3281] -> w3275
                    frame False {
                      # "We are not recording Step Value if it is linetrace"
                    }
                    frame True {
                      n2418 = flat-sequence {
                        tunnel: [w3285] -> w3280
                        tunnel: [w3284] -> w3279
                        tunnel: [w3283] -> w3278
                        frame #0 {
                          n2419 = property on="HandleOut" class="Clust (strict)"() -> ("Value"=w3288:T1)  [unwired: 2 in, 2 out]
                          n2420 = call "MFLIcontrol.vi"("MFLI function"=MFLIcommand."measure XY on demod3", "handle in"=w3288) -> ("Demod Sample Out 3"=w3286:T20)  [unwired: 5 in, 4 out]
                          n2421 = Unbundle(w3286) -> ("X (Vrms)"=w3285:dbl, "Y (Vrms)"=w3284:dbl, "Freq (Hz)"=w3283:dbl)  [unwired: 6 out]
                        }
                      }
                      n2422 = Build Array (concatenate)(w3282, w3280, w3279, w3278) -> (w3281:dbl[])
                    }
                  }
                  n2423 = property on="data" class="Arr (strict)"("Value"=w3275) -> ()  [unwired: 2 in, 2 out]
                }
                frame #55 {
                  # "Measure MFLI_I if \nit is checked"
                  n2424 = property on="MFLI2_d3" class="Bool (strict)"() -> ("Value"=w3289:bool)  [unwired: 2 in, 2 out]
                  n2425 = property on="data" class="Arr (strict)"() -> ("Value"=w3291:dbl[])  [unwired: 2 in, 2 out]
                  n2426 = case shown="True" w3289 {
                    tunnel: w3291 -> [w3292 w3297]
                    tunnel: [w3292 w3296] -> w3290
                    frame False {
                      # "We are not recording Step Value if it is linetrace"
                    }
                    frame True {
                      n2427 = flat-sequence {
                        tunnel: [w3300] -> w3295
                        tunnel: [w3299] -> w3294
                        tunnel: [w3298] -> w3293
                        frame #0 {
                          n2428 = property on="HandleOut 2" class="Clust (strict)"() -> ("Value"=w3303:T21)  [unwired: 2 in, 2 out]
                          n2429 = call "MFLIcontrol.vi"("MFLI function"=MFLIcommand."measure XY on demod3", "handle in"=w3303) -> ("Demod Sample Out 3"=w3301:T20)  [unwired: 5 in, 4 out]
                          n2430 = Unbundle(w3301) -> ("X (Vrms)"=w3300:dbl, "Y (Vrms)"=w3299:dbl, "Freq (Hz)"=w3298:dbl)  [unwired: 6 out]
                        }
                      }
                      n2431 = Build Array (concatenate)(w3297, w3295, w3294, w3293) -> (w3296:dbl[])
                    }
                  }
                  n2432 = property on="data" class="Arr (strict)"("Value"=w3290) -> ()  [unwired: 2 in, 2 out]
                }
                frame #56 {
                  # "Measure MFLI_I if \nit is checked"
                  n2433 = property on="MFLI3_d3" class="Bool (strict)"() -> ("Value"=w3304:bool)  [unwired: 2 in, 2 out]
                  n2434 = property on="data" class="Arr (strict)"() -> ("Value"=w3306:dbl[])  [unwired: 2 in, 2 out]
                  n2435 = case shown="True" w3304 {
                    tunnel: w3306 -> [w3307 w3312]
                    tunnel: [w3307 w3311] -> w3305
                    frame False {
                      # "We are not recording Step Value if it is linetrace"
                    }
                    frame True {
                      n2436 = flat-sequence {
                        tunnel: [w3315] -> w3310
                        tunnel: [w3314] -> w3309
                        tunnel: [w3313] -> w3308
                        frame #0 {
                          n2437 = property on="HandleOut 3" class="Clust (strict)"() -> ("Value"=w3318:T21)  [unwired: 2 in, 2 out]
                          n2438 = call "MFLIcontrol.vi"("MFLI function"=MFLIcommand."measure XY on demod3", "handle in"=w3318) -> ("Demod Sample Out 3"=w3316:T20)  [unwired: 5 in, 4 out]
                          n2439 = Unbundle(w3316) -> ("X (Vrms)"=w3315:dbl, "Y (Vrms)"=w3314:dbl, "Freq (Hz)"=w3313:dbl)  [unwired: 6 out]
                        }
                      }
                      n2440 = Build Array (concatenate)(w3312, w3310, w3309, w3308) -> (w3311:dbl[])
                    }
                  }
                  n2441 = property on="data" class="Arr (strict)"("Value"=w3305) -> ()  [unwired: 2 in, 2 out]
                }
                frame #57 {
                  # "Measure MFLI_I if \nit is checked"
                  n2442 = property on="MFLI4_d3" class="Bool (strict)"() -> ("Value"=w3319:bool)  [unwired: 2 in, 2 out]
                  n2443 = property on="data" class="Arr (strict)"() -> ("Value"=w3321:dbl[])  [unwired: 2 in, 2 out]
                  n2444 = case shown="True" w3319 {
                    tunnel: w3321 -> [w3322 w3327]
                    tunnel: [w3322 w3326] -> w3320
                    frame False {
                      # "We are not recording Step Value if it is linetrace"
                    }
                    frame True {
                      n2445 = flat-sequence {
                        tunnel: [w3330] -> w3325
                        tunnel: [w3329] -> w3324
                        tunnel: [w3328] -> w3323
                        frame #0 {
                          n2446 = property on="HandleOut 4" class="Clust (strict)"() -> ("Value"=w3333:T21)  [unwired: 2 in, 2 out]
                          n2447 = call "MFLIcontrol.vi"("MFLI function"=MFLIcommand."measure XY on demod3", "handle in"=w3333) -> ("Demod Sample Out 3"=w3331:T20)  [unwired: 5 in, 4 out]
                          n2448 = Unbundle(w3331) -> ("X (Vrms)"=w3330:dbl, "Y (Vrms)"=w3329:dbl, "Freq (Hz)"=w3328:dbl)  [unwired: 6 out]
                        }
                      }
                      n2449 = Build Array (concatenate)(w3327, w3325, w3324, w3323) -> (w3326:dbl[])
                    }
                  }
                  n2450 = property on="data" class="Arr (strict)"("Value"=w3320) -> ()  [unwired: 2 in, 2 out]
                }
                frame #58 {
                  # "Measure MFLI_I if \nit is checked"
                  n2451 = property on="MFLI1_AuxOut0" class="Bool (strict)"() -> ("Value"=w3334:bool)  [unwired: 2 in, 2 out]
                  n2452 = property on="data" class="Arr (strict)"() -> ("Value"=w3336:dbl[])  [unwired: 2 in, 2 out]
                  n2453 = case shown="True" w3334 {
                    tunnel: w3336 -> [w3337 w3340]
                    tunnel: [w3337 w3339] -> w3335
                    frame False {
                      # "We are not recording Step Value if it is linetrace"
                    }
                    frame True {
                      n2454 = flat-sequence {
                        tunnel: [w3341] -> w3338
                        frame #0 {
                          n2455 = property on="HandleOut" class="Clust (strict)"() -> ("Value"=w3343:T1)  [unwired: 2 in, 2 out]
                          n2456 = call "MFLIcontrol.vi"("MFLI function"=MFLIcommand."Get AuxOut0", "handle in"=w3343) -> ("AuxOut0_Ampl"=w3341:dbl)  [unwired: 5 in, 4 out]
                        }
                      }
                      n2457 = Build Array (concatenate)(w3340, w3338) -> (w3339:dbl[])
                    }
                  }
                  n2458 = property on="data" class="Arr (strict)"("Value"=w3335) -> ()  [unwired: 2 in, 2 out]
                }
              }
            }
            frame #4 {
              # "this part appends last\nmeasured point to the \ndata file"
              n2459 = local read "Data file:"() -> (w3345:path)
              n2460 = property on="data" class="Arr (strict)"() -> ("Value"=w3344:dbl[])  [unwired: 2 in, 2 out]
              n2461 = call-poly <vilib>:"Write To Spreadsheet File.vi"("format (%.3f)"="%.6e", "append to file? (new file:F)"=TRUE, "1D data"=w3344, "file path (dialog if empty)"=w3345) -> ()  [unwired: 4 in, 1 out]
            }
            frame #5 {
              n2462 = property on="data" class="Arr (strict)"() -> ("Value"=w3348:dbl[])  [unwired: 2 in, 2 out]
            }
          }
          n2463 = stacked-sequence "add data to array" {
            tunnel: w2538 -> [w3482]
            tunnel: [w3481] -> w2537
            tunnel: w2524 -> [w3480]
            frame #0 {
              n2464 = Build Array (concatenate)(w3482, w3480) -> (w3481:dbl[][])
            }
          }
          n2465 = And(x=w2526, y="Continuous Sweep") -> (x .and. y?=w2530:bool)
          n2466 = case shown="True" w2530 {
            frame False {
            }
            frame True {
              n2467 = property on="upper limit" class="DigNum (strict)"() -> ("Value"=w2539:dbl)  [unwired: 2 in, 2 out]
              n2468 = local read "sweep to:"() -> (w2541:dbl)
              n2469 = property on="lower limit" class="DigNum (strict)"() -> ("Value"=w2540:dbl)  [unwired: 2 in, 2 out]
              n2470 = Equal?(x=w2541, y=w2539) -> (x = y?=w2542:bool)
              n2471 = Select(t=w2540, s=w2542, f=w2539) -> (s? t:f=w2543:dbl)
              n2472 = local write "sweep to:"(w2543) -> ()
            }
          }
          n2473 = stacked-sequence "plot selected measurements" {
            seq-local: [_ w3505 _] -> [_ _ w3550]
            seq-local: [_ w3504 _] -> [_ _ w3551]
            tunnel: w2537 -> [_ w3503 _]
            frame #0 {
              n2474 = property on="XY Graph" class="XYGraph (strict)"("ActYScl"=0 ("Active Y Scale")) -> (error out=w3488:errorcluster)  [unwired: 2 in, 1 out]
              n2475 = property on="Show cursor" class="Bool (strict)"() -> ("Value"=w3483:bool)  [unwired: 2 in, 2 out]
              n2476 = property on="Xaxis" class="Ring (strict)"() -> ("Value"=w3493:u16)  [unwired: 2 in, 2 out]
              n2477 = property on="Yaxis" class="Ring (strict)"(error in=w3488) -> (error out=w3487:errorcluster, "RingText.Text"=w3486:string)  [unwired: 1 in, 1 out]
              n2478 = property on="XY Graph" class="XYGraph (strict)"("Cursor.Visible"=w3483) -> ()  [unwired: 2 in, 2 out]
              n2479 = property on="Figure_axis" class="Arr (strict)"() -> ("Value"=w3494:string[])  [unwired: 2 in, 2 out]
              n2480 = property on="XY Graph" class="XYGraph (strict)"(error in=w3487, "YScale.NameLbl.Text"=w3486) -> (error out=w3484:errorcluster)  [unwired: 1 in, 1 out]
              n2481 = property on="XY Graph" class="XYGraph (strict)"(error in=w3484, "ActYScl"=1 ("Active Y Scale")) -> (error out=w3490:errorcluster)  [unwired: 1 in, 1 out]
              n2482 = property on="Yright" class="Ring (strict)"(error in=w3490) -> (error out=w3491:errorcluster, "RingText.Text"=w3485:string)  [unwired: 1 in, 1 out]
              n2483 = Index Array(array=w3494, index=w3493) -> (element=w3495:string)
              n2484 = property on="XY Graph" class="XYGraph (strict)"("XScale.NameLbl.Text"=w3495) -> ()  [unwired: 2 in, 2 out]
